vi "App - analyze RUS V6.vi"() -> ()   [LabVIEW 2015] (continued)
      w53 = FALSE  # Visible
      n14 = local read "parameters: wavepacket"() -> (w56:T16)
      n15 = local write "in sweep folder"(w57) -> ()
      n16 = call "follow the peak controller.vi"("action"=follow_the_peak_action."follow the peak", "follow the peak ref"=w50) -> ()  [unwired: 8 in, 2 out]
      n17 = property on="-- loading ..." class="Bool (strict)"("Visible"=w53) -> ()  [unwired: 2 in, 2 out]
      n18 = property on="back to temperature folder" class="Bool"("Visible"=w53) -> ()  [unwired: 2 in, 2 out]
      n19 = Bundle By Name(cluster=w56, "wavepacket is"=w52) -> (w55:T16)
      n20 = local write "parameters: wavepacket"(w55) -> ()
    }
  }
  n21 = register-events(w16, w18) -> (reference out=w48:refnum<event-registration>)  [unwired: 2 in, 1 out]
  n22 = control-ref of="save/read"() -> (w1:refnum<vi>)
  n23 = control-ref of="cursor bracket: All,  show"() -> (w19:refnum<vi>)
  n24 = control-ref of="cursor bracket: All, data window"() -> (w24:refnum<vi>)
  n25 = control-ref of="cursor bracket: All,  zoom"() -> (w23:refnum<vi>)
  n26 = control-ref of="cursor bracket: fragment"() -> (w25:refnum<vi>)
  n27 = control-ref of="cursor bracket: Time"() -> (w22:refnum<vi>)
  n28 = control-ref of="Plot: Time"() -> (w21:refnum<vi>)
  n29 = control-ref of="Plot: All"() -> (w20:refnum<vi>)
  n30 = control-ref of="Plot: fragment"() -> (w26:refnum<vi>)
  n31 = Create User Event(user event datatype=w34) -> (user event=w33:refnum<user-event>)  [unwired: 1 in, 1 out]
  n32 = Create User Event(user event datatype=w32) -> (user event=w17:refnum<user-event>)  [unwired: 1 in, 1 out]
  n33 = Create User Event(user event datatype=w47) -> (user event=w44:refnum<user-event>)  [unwired: 1 in, 1 out]
  n34 = while {
    tunnel: w48 -> [w72]
    tunnel: w16 -> [w70]
    tunnel: w44 -> [w69]
    tunnel: w36 -> [_]
    tunnel: w18 -> [w64]
    tunnel: w33 -> [w63]
    tunnel: w17 -> [w61]
    tunnel: w6 -> [w60]
    tunnel: w1 -> [w58]
    i -> [w62]
    stop <- FALSE stop-if-true
    n35 = Wait (ms)(milliseconds to wait=u32 2) -> ()  [unwired: 1 out]
    n36 = Equal To 0?(x=w62) -> ()  [unwired: 1 out]
    n37 = control-ref of="follow the peak"() -> (w59:refnum<vi>)
    n38 = event shown="[0] <calculate>: User Event" {
      selector: w72 -> [_ _ _ _ _ _ _ _ _ _]
      dyn-events: _ -> [_ _ _ _ _ _ _ _ _ _]
      timeout: 1 -> [_ _ _ _ _ _ _ _ _ _]
      tunnel: w70 -> [w98 w515 _ _ _ _ _ _ w1074 _]
      tunnel: w69 -> [_ _ _ _ _ _ _ _ _ _]
      tunnel: [_ _ _ "back to temperature folder" _ _ _ _ _ _] -> _
      tunnel: TRUE -> [w97 _ _ _ _ _ _ _ _ _]
      tunnel: FALSE -> [_ w517 _ _ w1054 _ _ _ _ _]
      tunnel: w64 -> [w100 w516 w1040 _ w1059 w1068 w1072 _ w1081 _]
      tunnel: [_ _ "Sweep folder path" _ _ _ _ _ _ _] -> _
      tunnel: w63 -> [w89 w513 _ _ _ _ _ _ _ _]
      tunnel: w61 -> [_ w491 w1038 _ _ _ _ _ _ _]
      tunnel: w60 -> [w75 _ _ _ _ _ _ _ _ _]
      tunnel: w59 -> [_ w488 _ _ _ _ _ _ _ _]
      tunnel: w58 -> [_ _ _ _ w1053 w1065 w1069 _ _ _]
      event User Event {
        w84 = FALSE  # scan/single peak
        # "all z"
        # "all omega"
        n39 = event-data() -> ("calculate"=w99:string)  [unwired: 1 in]
        n40 = local read "Sweep folder path"() -> (w81:path)
        n41 = local read "parameters: center detection"() -> (w91:T21)
        n42 = control-ref of="cursor bracket: All, data window"() -> (w95:refnum<vi>)
        n43 = local read "parameters: wavepacket"() -> (w93:T16)
        n44 = local read "parameters: omega map"() -> (w88:T22)
        n45 = local read "temperature(K)"() -> (w82:dbl)
        n46 = local read "follow the peak"() -> (w74:T7)
        n47 = control-ref of="cursor bracket: fragment"() -> (w94:refnum<vi>)
        n48 = local read "in sweep folder"() -> (w83:bool)
        n49 = local read "complex region"() -> (w90:T25)
        n50 = control-ref of="slide control"() -> (w73:refnum<vi>)
        n51 = local read "file path"() -> (w92:path)
        n52 = control-ref of="cursor bracket: All,  zoom"() -> ()  [unwired: 1 out]
        n53 = control-ref of="Plot: All"() -> (w85:refnum<vi>)
        n54 = control-ref of="cursor bracket: All,  show"() -> (w86:refnum<vi>)
        n55 = local read "plot filter progress?"() -> (w78:bool)
        n56 = Current VI's Path "Current VI's Path (this allows to inline fit function)"() -> (path=w87:path)
        n57 = control-ref of="Plot: fragment filter"() -> (w80:refnum<vi>)
        n58 = control-ref of="Plot: complex plane - filter"() -> (w79:refnum<vi>)
        n59 = for {
          N: 1 -> [_]
          tunnel: w100 -> [w131]
          tunnel: w99 -> [w130]
          tunnel: w98 -> [w129]
          tunnel: w97 -> [w126]
          shift-right: [w125] -> _
          shift-left: _ -> [w128]
          shift-right: [w124] -> _
          shift-left: _ -> [w127]
          tunnel: w95 -> [w123]
          tunnel: w94 -> [w122]
          tunnel: w93 -> [w121]
          tunnel: w92 -> [w120]
          tunnel: w91 -> [w119]
          tunnel: w90 -> [w118]
          tunnel: w89 -> [w117]
          tunnel: w88 -> [w116]
          tunnel: w87 -> [w115]
          tunnel: w86 -> [w114]
          tunnel: w85 -> [w113]
          tunnel: w84 -> [w112]
          tunnel: w83 -> [w111]
          tunnel: w82 -> [w110]
          tunnel: w81 -> [w109]
          tunnel: w80 -> [w108]
          tunnel: w79 -> [w107]
          tunnel: w78 -> [w106]
          tunnel: "filter method" -> [w105]
          tunnel: "parameters: complex fit" -> [w104]
          tunnel: w75 -> [w103]
          tunnel: w74 -> [w102]
          tunnel: w73 -> [w101]
          n60 = case shown="\"calc:peak\"" w130 {
            tunnel: w131 -> [_ _ _ w275 _ _]
            tunnel: w129 -> [_ w162 _ w268 _ w443]
            tunnel: w128 -> [w142 w151 w240 w274 w363 _]
            tunnel: w127 -> [w141 w152 w239 w273 w371 _]
            tunnel: w126 -> [_ _ _ _ _ _]
            tunnel: [w142 w151 w240 w274 w363 w442] -> w125
            tunnel: [w141 w152 w239 w273 w371 w441] -> w124
            tunnel: w123 -> [_ w148 w238 w269 w361 _]
            tunnel: w122 -> [_ _ _ w263 _ _]
            tunnel: w121 -> [w134 _ _ w264 w374 _]
            tunnel: w120 -> [_ _ _ _ _ w440]
            tunnel: w119 -> [w135 w161 _ w272 _ _]
            tunnel: w118 -> [_ _ _ _ _ _]
            tunnel: w117 -> [_ w160 _ w271 w359 _]
            tunnel: w116 -> [_ _ _ w266 _ _]
            tunnel: w115 -> [_ _ _ w270 w368 _]
            tunnel: w114 -> [_ _ _ _ w367 _]
            tunnel: w113 -> [_ _ _ w267 w353 _]
            tunnel: w112 -> [_ _ _ _ _ _]
            tunnel: w111 -> [_ _ _ w265 w360 _]
            tunnel: w110 -> [_ _ _ _ w356 _]
            tunnel: w109 -> [_ _ w218 _ _ _]
            tunnel: w108 -> [_ w159 _ _ _ _]
            tunnel: w107 -> [_ w158 _ _ _ _]
            tunnel: w106 -> [_ w157 _ _ _ _]
            tunnel: w105 -> [_ w156 _ _ _ _]
            tunnel: w104 -> [_ w143 _ w262 _ _]
            tunnel: w103 -> [_ w144 _ w261 _ _]
            tunnel: w102 -> [_ _ _ w260 _ _]
            tunnel: w101 -> [_ _ _ _ _ w435]
            frame "calc:wavepacket", Default {
              n61 = call "single fit V5.vi"("single fit parameters"=w135, "find fit action"=find_peak_action."update pond", "parameters: wavepacket"=w134) -> ("parameters: wavepacket  out"=w132:T16)  [unwired: 8 in, 4 out]
              n62 = Unbundle By Name(w132) -> ("radii vector"=w138:dbl[], "radial section"=w139:cdb[])
              n63 = Complex To Re/Im(x + iy=w139) -> (x=w137:dbl[])  [unwired: 1 out]
              n64 = local write "parameters: wavepacket"(w132) -> ()
              n65 = Bundle("radii vector"=w138, w137) -> (w136:cluster{"radii vector":dbl[], dbl[]})  [unwired: 1 in]
              n66 = Build Array(w136) -> (→"Plot: wavepacket":cluster{"radii vector":dbl[], dbl[]}[])
            }
            frame "calc:new cursor bracket" {
              n67 = call "cursor window logic V2.vi"("cursor window action"=cursor_window_action."check", "cursor window in"=w148) -> ("cursor window out"=w154:T24)  [unwired: 8 in, 1 out]
              n68 = Unbundle By Name(w154) -> ("window"=→"window":dbl)
              n69 = call "acquire cursor window data.vi"("z in"=w152, "omega in"=w151, "cursor window"=w154) -> ("z out"=w149:cdb[], "omega  out"=w150:dbl[])  [unwired: 4 in, 3 out]
              n70 = Array Size(array=w150) -> (size(s)=w147:i32)
              "# points" <- w147
              n71 = Greater?(x=w147, y=15) -> (0:w146:bool)
              n72 = case shown="True" w146 {
                tunnel: w162 -> [_ w174]
                tunnel: w161 -> [_ w173]
                tunnel: w160 -> [_ w172]
                tunnel: w159 -> [_ w171]
                tunnel: w158 -> [_ w170]
                tunnel: w157 -> [_ w169]
                tunnel: w156 -> [_ w168]
                tunnel: w150 -> [_ w167]
                tunnel: w149 -> [_ w166]
                tunnel: w144 -> [_ w165]
                tunnel: w143 -> [_ w164]
                tunnel: w143 -> [_ w163]
                frame False {
                }
                frame True {
                  n73 = flat-sequence {
                    tunnel: w173 -> [w192]
                    tunnel: w171 -> [_]
                    tunnel: w170 -> [_]
                    tunnel: w169 -> [w186]
                    tunnel: w168 -> [w185]
                    tunnel: w167 -> [w184]
                    tunnel: w166 -> [w183]
                    tunnel: w165 -> [w182]
                    tunnel: w164 -> [w181]
                    tunnel: w163 -> [_]
                    tunnel: w174 -> [w211]
                    tunnel: w172 -> [w210]
                    tunnel: [w208] -> _
                    frame #0 {
                      (unwired) TRUE
                      n74 = call "filter - complex - four.vi"("omega  in"=w184, "z in"=w183, "span"="smart filter: span", "filter method"=w185) -> ("center"=w189:cdb, "norm"=w188:dbl, "omega out"=w179:dbl[], "z in out"=w190:cdb[], "z out"=w178:cdb[], "win omega out"=w180:dbl[], "dz/domega out"=w177:cdb[], "tale of three"=w191:T38)  [unwired: 8 in]
                      "complex plane center" <- w189
                      "complex plane norm" <- w188
                      n75 = call "peak -- PM find lorenzian - V2.vi"("omega"=w179, "z"=w178, "dz/domega"=w177) -> ("phase (around center)"=w175:dbl[], "poor man lorentzian"=w176:T11)  [unwired: 9 in, 2 out]
                      n76 = case shown="True" w186 {
                        tunnel: w191 -> [_ w205]
                        tunnel: w190 -> [_ w204]
                        tunnel: w189 -> [_ w203]
                        tunnel: w188 -> [_ w202]
                        tunnel: w179 -> [_ w201]
                        tunnel: w178 -> [_ w200]
                        tunnel: w182 -> [_ w199]
                        tunnel: w181 -> [_ w198]
                        tunnel: w177 -> [_ w197]
                        tunnel: w180 -> [_ w196]
                        tunnel: w176 -> [_ w195]
                        tunnel: w175 -> [_ w194]
                        frame False {
                        }
                        frame True {
                          n77 = call "filter pipe - plot staff - more - V2.vi"("omega  in"=w201, "zin"=w204, "z out"=w200, "win omega"=w196, "phase"=w194, "dz/domega in"=w197, "center"=w203, "plots: filter related"=w199, "norm"=w202, "parameters: complex fit"=w198, "tale of three indices -- int -- control"=w205, "lorentzian"=w195) -> ()  [unwired: 8 in]
                        }
                      }
                      n78 = Bundle By Name(cluster=w192, "dz/domega"=w177, "omega in window"=w179, "z in window"=w178) -> (w193:T21)
                      n79 = local write "parameters: center detection"(w193) -> ()
                    }
                    frame #1 {
                      # "attempts at optimization :\nsmall arrays are in variables\nlarge arrays are in shift registers"
                      # "send recalculate"
                      n80 = Generate User Event(user event=w211, event data cluster="calc:peak" ("event data")) -> (error out=w209:errorcluster)  [unwired: 2 in, 1 out]
                      n81 = case shown="True" TRUE {
                        tunnel: w210 -> [_ w216]
                        tunnel: w209 -> [w212 w214]
                        tunnel: [w212 w213] -> w208
                        frame False {
                        }
                        frame True {
                          n82 = Generate User Event(user event=w216, event data cluster="check fragment zoom" ("event data"), error in=w214) -> (error out=w213:errorcluster)  [unwired: 1 in, 1 out]
                        }
                      }
                    }
                  }
                }
              }
              n83 = disable-structure shown="Disabled" {
                frame Disabled {
                  n84 = local read "interpolated gamma"() -> ()  [unwired: 1 out]
                  n85 = local read "interpolated omega"() -> ()  [unwired: 1 out]
                  n86 = local read item#-1() -> ()  [unwired: 1 out]
                }
                frame Enabled {
                }
              }
            }
            frame "save cursor window" {
              w228 = "kHz_"
              n87 = call "file -- 9w path.vi"("sweep folder"=w218) -> ("9w path"=w217:path)  [unwired: 10 in]
              n88 = call "cursor window logic V2.vi"("cursor window action"=cursor_window_action."check", "cursor window in"=w238) -> ("cursor window out"=w233:T24)  [unwired: 8 in, 1 out]
              n89 = call "acquire cursor window data.vi"("z in"=w239, "omega in"=w240, "cursor window"=w233) -> ("z out"=w222:cdb[], "omega  out"=w223:dbl[])  [unwired: 4 in, 3 out]
              n90 = Unbundle By Name(w233) -> ("left"=w232:dbl, "right"=w231:dbl)
              n91 = Number To Decimal String(number=w232) -> (decimal integer string=w230:string)  [unwired: 1 in]
              n92 = Number To Decimal String(number=w231) -> (decimal integer string=w229:string)  [unwired: 1 in]
              n93 = for {
                tunnel: w223 -> [w245] mode=indexing
                tunnel: w222 -> [w242] mode=indexing
                tunnel: [w241] -> w221 mode=indexing
                n94 = Complex To Re/Im(x + iy=w242) -> (x=w244:dbl, y=w243:dbl)
                n95 = Format Into String(format string="%f\\t%f\\t%f", w245, w244, w243) -> (resulting string=w241:string)  [unwired: 2 in, 1 out]
              }
              n96 = Strip Path(path=w217) -> (stripped path=w237:path, name=w236:string)
              n97 = call "Split file name.vi"("file name"=w236) -> ("name"=w234:string)  [unwired: 8 in, 2 out]
              n98 = Concatenate Strings(w234, "_cursor_", w230, w228, w229, w228, ".dat") -> (w226:string)
              n99 = Build Path(base path=w237, name or relative path=w226) -> (appended path=w220:path)
              n100 = call-poly <vilib>:"Write To Spreadsheet File.vi"("delimiter (\\t)"="\r", "append to file? (new file:F)"=FALSE, "1D data"=w221, "file path (dialog if empty)"=w220) -> ()  [unwired: 4 in, 1 out]
            }
            frame "calc:peak" {
              (unwired) 1
              n101 = flat-sequence {
                tunnel: w261 -> [w277]
                tunnel: w262 -> [w278]
                tunnel: w264 -> [w279]
                tunnel: w269 -> [w280]
                tunnel: w266 -> [w281]
                tunnel: w272 -> [w282]
                tunnel: [w282] -> w257
                tunnel: [w281] -> w256
                tunnel: [w280] -> w255
                tunnel: [w279] -> w254
                tunnel: [w278] -> w253
                tunnel: [w277] -> w252
                tunnel: [w276] -> w250
                tunnel: w270 -> [_]
                tunnel: w263 -> [w295]
                tunnel: w267 -> [w299]
                tunnel: [w294] -> w259
                tunnel: w260 -> [w289]
                tunnel: w257 -> [w304]
                tunnel: w256 -> [w301]
                tunnel: w255 -> [w298]
                tunnel: w254 -> [w292]
                tunnel: w253 -> [w291]
                tunnel: w252 -> [w290]
                tunnel: [w286] -> w251
                tunnel: w250 -> [w286]
                tunnel: "Use C++" -> [w285]
                tunnel: "find fit action" -> [w284]
                tunnel: "plot pm ?" -> [w283]
                tunnel: w259 -> [w334]
                tunnel: [w334] -> w258
                tunnel: w251 -> [w332]
                tunnel: w275 -> [w341]
                tunnel: w265 -> [w340]
                tunnel: w271 -> [w339]
                tunnel: w268 -> [w338]
                tunnel: w258 -> [w335]
                frame #0 {
                  n102 = Tick Count (ms)() -> (millisecond timer value=w276:u32)
                }
                frame #1 {
                  n103 = case shown="True" w285 {
                    tunnel: w304 -> [w317 w330]
                    tunnel: [w316 w329] -> w303
                    tunnel: [w315 w328] -> w302
                    tunnel: w301 -> [w314 w327]
                    tunnel: [w313 w326] -> w300
                    tunnel: [w312 w325] -> w297
                    tunnel: w295 -> [w311 w324]
                    tunnel: w284 -> [w310 w323]
                    tunnel: [w309 w322] -> w293
                    tunnel: w292 -> [w308 w321]
                    tunnel: w291 -> [w307 w320]
                    tunnel: w290 -> [w306 w319]
                    tunnel: w283 -> [w305 w318]
                    frame True {
                      n104 = call "single fit V5cpp.vi"("single fit parameters"=w317, "plot what"=w305, "find fit action"=w310, "cursor bracket: fragment  ref"=w311, "omega map parameters"=w314, "parameters: wavepacket"=w308, "parameters: complex fit"=w307, "plots: filter related"=w306) -> ("single fit parameters out"=w316:T21, "omega map parameters out"=w315:T22, "parameters: wavepacket  out"=w309:T16, "complex region out"=w313:T25, "lorentzian out"=w312:T11)  [unwired: 3 in]
                    }
                    frame False {
                      n105 = call "single fit V5.vi"("single fit parameters"=w330, "plot what"=w318, "find fit action"=w323, "cursor bracket: fragment  ref"=w324, "omega map parameters"=w327, "parameters: wavepacket"=w321, "parameters: complex fit"=w320, "plots: filter related"=w319) -> ("single fit parameters out"=w329:T21, "omega map parameters out"=w328:T22, "parameters: wavepacket  out"=w322:T16, "complex region out"=w326:T25, "lorentzian out"=w325:T11)  [unwired: 3 in]
                    }
                  }
                  n106 = local write "parameters: center detection"(w303) -> ()
                  n107 = local write "parameters: wavepacket"(w293) -> ()
                  n108 = local write "parameters: omega map"(w302) -> ()
                  n109 = call "shake it.vi"("cursor bracket : fragment 2"=w295, "cursor bracket: All, data window 2"=w298, "Plot: All"=w299, "follow the peak Con"=w289, "search attempts"=4, "peak close to center -- factor"=0.3, "lorentzian"=w297) -> ("Boolean"=w294:bool, "lorentzian out"=w296:T11)  [unwired: 1 in, 2 out]
                  n110 = local write "complex region"(w300) -> ()
                  n111 = local write "lorentzian"(w296) -> ()
                }
                frame #2 {
                  n112 = Tick Count (ms)() -> (millisecond timer value=w333:u32)
                  n113 = Subtract(x=w333, y=w332) -> (x-y=→"fit time (ms)":u32)
                }
                frame #3 {
                  n114 = case shown="True" w335 {
                    tunnel: w341 -> [_ w348]
                    tunnel: w340 -> [_ w347]
                    tunnel: w339 -> [_ w346]
                    tunnel: w338 -> [w343 _]
                    tunnel: [w343 w345] -> w337
                    tunnel: ["calc:new cursor bracket" ("t.folder") w344] -> w336
                    frame False {
                    }
                    frame True {
                      n115 = case shown="True" w347 {
                        tunnel: w348 -> [_ w352]
                        tunnel: w346 -> [w350 _]
                        tunnel: [w350 w352] -> w345
                        tunnel: ["calculation finished" ("t.folder") "update freq/atten" ("t.folder")] -> w344
                        frame False {
                        }
                        frame True {
                        }
                      }
                    }
                  }
                  n116 = Generate User Event(user event=w337, event data cluster=w336) -> ()  [unwired: 2 in, 2 out]
                }
              }
            }
            frame "calc: scan" {
              n117 = property class="Clust (strict)"(reference=w361) -> ("Value"=w366:T39)  [unwired: 1 in, 2 out]
              n118 = Unbundle By Name(w366) -> ("left"=w365:dbl, "right"=w364:dbl)
              n119 = Array Size(array=w371) -> (size(s)=w373:i32)
              n120 = call "index from range.vi"("left"=w365, "right"=w364, "omega"=w363) -> ("length"=w362:dbl)  [unwired: 6 in, 2 out]
              n121 = Quotient & Remainder(x=w373, y="scan speed") -> (floor(x/y)=w372:i32)  [unwired: 1 out]
              n122 = for {
                N: w372 -> [_]
                tunnel: w374 -> [w425]
                tunnel: w363 -> [w423]
                tunnel: w371 -> [w433]
                shift-right: [w422] -> _
                shift-left: 0 -> [w414]
                tunnel: "scan speed" -> [w432]
                tunnel: w368 -> [w431]
                tunnel: w367 -> [_]
                tunnel: w353 -> [w416]
                tunnel: w362 -> [w411]
                tunnel: w361 -> [w412]
                tunnel: [w405] -> w357
                tunnel: "number of hits to threshold" -> [w407]
                tunnel: "threshold window" -> [w406]
                i -> [w434]
                n123 = Add(x=w414, y=w432) -> (x+y=w422:i32)
                n124 = Equal To 0?(x=w434) -> (x = 0?=w408:bool)
                n125 = Subtract(x=w414, y=w411) -> (x-y=w413:dbl)
                n126 = Array Subset(array=w423, index=w414, length=w432) -> (w429:dbl[])
                n127 = Index Array(array=w423, index #1=w414, index #2=w413) -> (element #1=w421:dbl, element #2=w420:dbl)
                n128 = Array Subset(array=w433, index=w414, length=w432) -> (w430:cdb[])
                n129 = Subtract(x=w420, y=w421) -> ()  [unwired: 1 out]
                n130 = Add(x=w421, y=w420) -> (x+y=w419:dbl)
                n131 = Divide(x=w419, y=2) -> (x/y=w409:dbl)
                n132 = call "curvature-cator - ia.vi"("omega array in"=w429, "size"=w411, "number of grid points"=70, "decimation threshold"=1, "z array in"=w430, "wavepacket in"=w425, "scale factor"=3.0, "first time"=w408, "main VI path"=w431) -> ("lorentzian out"=w424:T11)  [unwired: 3 in, 3 out]
                n133 = call "cursor window logic V2.vi"("cursor window action"=cursor_window_action."change center", "center"=w409, "cursor window in"=w412) -> ("cursor window out"=w403:T24)  [unwired: 7 in, 1 out]
                n134 = Unbundle By Name(w424) -> ("omega(0)"=w396:dbl)  [unwired: 1 out]
                n135 = call "aggregator - i.vi"("requested averaging interval"=10, "first time"=w408, "requested size"=w411, "number"=w396) -> ()  [unwired: 3 in, 5 out]
                n136 = call "aggregator - i.vi"("first time"=w408, "requested size"=w411, "number"=w409) -> ()  [unwired: 4 in, 5 out]
                n137 = Unbundle By Name(w403) -> ("left"=w402:dbl, "right"=w401:dbl)
                n138 = call "Q -- check range.vi"("upper"=w401, "lower"=w402, "number"=w396) -> ("in range?"=w397:bool)  [unwired: 4 in, 4 out]
                n139 = Select(t=w396, s=w397, f=nan ("scale factor")) -> (s? t:f=w394:dbl)
                n140 = call "threshold-icator - i.vi"("first time"=w408, "requested size"=w407, "gamma"=w406, "omega"=w394) -> ("new peak"=w393:bool, "array of peaks"=w405:dbl[])  [unwired: 3 in, 3 out]
                "array of peaks" <- w405
                n141 = Select(t=u32 327424 ("Color Box"), s=w393, f=u32 16716367 ("Color Box")) -> (s? t:f=w398:u32)
                n142 = call "replace cursor - plot ref.vi"("cursor state"=T35."colored", "Color Box"=w398, "action"=enum16{"", "read", "write"}."write" ("Enum"), "cursor index"=9, "new X"=w396, "Plot ref in"=w416) -> ()  [unwired: 3 in, 3 out]
              }
              n143 = case shown="True" w360 {
                selector: w360 -> [_ w379]
                tunnel: w359 -> [_ w385]
                tunnel: "calculation finished" ("t.folder") -> [_ w384]
                tunnel: w357 -> [_ w383]
                tunnel: w356 -> [_ w382]
                frame False {
                }
                frame True {
                  n144 = call "switch - C.vi"("switch"=w379) -> ("result"=w378:bool)  [unwired: 10 in]
                  n145 = for {
                    tunnel: w383 -> [w391] mode=indexing
                    tunnel: w382 -> [w390]
                    tunnel: [w389] -> w376
                    tunnel: [w388] -> w375
                    tunnel: w378 -> [w387]
                    tunnel: 50000 -> [w386]
                    n146 = call "aggregator.vi"("first time"=w387, "requested size"=w386, "number"=w390) -> ("Array"=w388:cdb[])  [unwired: 8 in]
                    n147 = call "aggregator.vi"("first time"=w387, "requested size"=w386, "number"=w391) -> ("Array"=w389:cdb[])  [unwired: 8 in]
                  }
                  n148 = Bundle("Array"=w375, "Array"=w376) -> (w381:cluster{"Array":cdb[], "Array":cdb[]})  [unwired: 1 in]
                  n149 = Build Array(w381) -> (→"Plot: JBBetts":cluster{"Array":cdb[], "Array":cdb[]}[])
                  n150 = Generate User Event(user event=w385, event data cluster=w384) -> ()  [unwired: 2 in, 2 out]
                }
              }
            }
            frame "calc:new file" {
              n151 = flat-sequence {
                tunnel: w440 -> [w447]
                tunnel: [w447] -> w439
                tunnel: [w446] -> w437
                tunnel: [w463] -> w445
                tunnel: [w462] -> w444
                tunnel: w439 -> [w464]
                tunnel: w435 -> [w451]
                tunnel: [w483] -> w441
                tunnel: [w484] -> w442
                tunnel: w445 -> [w484]
                tunnel: w444 -> [w483]
                tunnel: w443 -> [w482]
                tunnel: [w480] -> w438
                frame #0 {
                  n152 = Tick Count (ms)() -> (millisecond timer value=w446:u32)
                }
                frame #1 {
                  # "Hz/kHz"
                  n153 = local read "plot fit progress?"() -> (w457:bool)
                  n154 = call "slide controller.vi"("slide action"=slide_action."check", "slide control"=w451) -> ("in slide"=w449:bool)  [unwired: 6 in, 3 out]
                  n155 = Not(x=w457) -> (.not. x?=w459:bool)
                  n156 = And(x=w459, y=w449) -> (x .and. y?=w458:bool)
                  n157 = call "rus fit - load data file.vi"("file path"=w464, "read scan file"="read scan file options") -> ("all:max omega"=→"all:max omega":dbl, "all:min omega"=→"all:min omega":dbl, "omega"=w463:dbl[], "x + iy"=w462:cdb[])  [unwired: 5 in, 1 out]
                  n158 = Not(x=w458) -> (.not. x?=w456:bool)
                  n159 = control-ref of="Plot: All"() -> (w453:refnum<vi>)
                  n160 = case shown="True" w456 {
                    tunnel: w463 -> [_ w474]
                    tunnel: w462 -> [_ w473]
                    frame False {
                    }
                    frame True {
                      n161 = Complex To Re/Im(x + iy=w473) -> (x=w476:dbl[], y=w475:dbl[])
                      n162 = Bundle("omega"=w474, w476) -> (w477:cluster{"omega":dbl[], dbl[]})  [unwired: 1 in]
                      n163 = Bundle("omega"=w474, w475) -> (w478:cluster{"omega":dbl[], dbl[]})  [unwired: 1 in]
                      n164 = Build Array(w477, w478) -> (→"Plot: All":cluster{"omega":dbl[], dbl[]}[])
                    }
                  }
                  n165 = case shown="\"log-log\"" "mapping: All" {
                    tunnel: [u8 0 ("X Scale.Mapping Mode") u8 1 ("X Scale.Mapping Mode") u8 0 ("X Scale.Mapping Mode") u8 1 ("X Scale.Mapping Mode")] -> w455
                    tunnel: [u8 0 ("X Scale.Mapping Mode") u8 0 ("X Scale.Mapping Mode") u8 1 ("X Scale.Mapping Mode") u8 1 ("X Scale.Mapping Mode")] -> w452
                    frame "linear-linear", Default {
                    }
                    frame "log-linear" {
                    }
                    frame "linear-log" {
                    }
                    frame "log-log" {
                    }
                  }
                  n166 = property on="Property Node" class="XYGraph (strict)"(reference=w453, "XScale.Mapping Mode"=w455, "YScale.Mapping Mode"=w452) -> ()  [unwired: 1 in, 2 out]
                }
                frame #2 {
                  n167 = Tick Count (ms)() -> (millisecond timer value=w480:u32)
                  n168 = Generate User Event(user event=w482, event data cluster="calc:new cursor bracket" ("event data")) -> ()  [unwired: 2 in, 2 out]
                }
              }
              n169 = Subtract(x=w438, y=w437) -> (x-y=→"ms per read":u32)
            }
          }
        }
      }
      event User Event {
        # "Temperature folder logic:\nwe load the whole folder (temperatures, timestamps,  paths -- not the data) in \"sweep folder file path array\".\nFiles are  navigated by using \"time (min)\" variable. The lorentzian fits are stored in \n\"frequency points\", \"attenuation points\" etc arrays and are displayed in plots.\n\nWhen we read a single file the variable \"in temperature folder\" is FALSE  and nothing of the above (and below) applies"
        n170 = event-data() -> ("temperature folder control"=w510:string)  [unwired: 1 in]
        n171 = local read "t.folder file path array"() -> (w499:T26[])
        n172 = local read "cursor bracket: Time"() -> (w502:T24)
        n173 = local read "temperature points"() -> (w500:dbl[])
        n174 = local read "best fit parameters"() -> (w494:dbl[])
        n175 = local read "attenuation points"() -> (w486:dbl[])
        n176 = local read "Sweep folder path"() -> (w511:path)
        n177 = local read "Magn Field points"() -> (w485:dbl[])
        n178 = local read "frequency points"() -> (w490:dbl[])
        n179 = local read "lorentzian points"() -> (w497:T27[])
        n180 = local read "in sweep folder"() -> (w509:bool)
        n181 = local read "9w folder path"() -> (w505:path)
        n182 = local read "time points"() -> (w501:dbl[])
        n183 = local read "lorentzian"() -> (w503:T11)
        n184 = local read "file path"() -> (w504:path)
        n185 = local read "fit using"() -> (w493:T5)
        n186 = control-ref of="Plot: Time"() -> (w496:refnum<vi>)
        n187 = local read "tfolder"() -> (w498:T30)
        n188 = control-ref of="cursor bracket: Time"() -> (w489:refnum<vi>)
        n189 = control-ref of="save/read"() -> (w487:refnum<vi>)
        n190 = control-ref of="cursor bracket: Time"() -> (w508:refnum<vi>)
        n191 = control-ref of="cursor bracket: All, data window"() -> (w507:refnum<vi>)
        n192 = control-ref of="cursor bracket: All,  zoom"() -> ()  [unwired: 1 out]
        n193 = control-ref of="cursor bracket: fragment"() -> (w506:refnum<vi>)
        n194 = case shown="\"new temperature folder\"" w510 {
          tunnel: w511 -> [w521 _ _ _ _ _ w690 w715 _ _ _ _ _ _ _ _ _]
          tunnel: TRUE -> [w530 _ _ _ _ _ _ w709 _ _ _ _ _ _ _ _ _]
          tunnel: w517 -> [_ _ _ _ _ _ _ _ _ w821 _ _ _ _ _ _ _]
          tunnel: w516 -> [_ _ _ _ w581 _ _ w720 _ _ _ _ w994 _ _ _ w1028]
          tunnel: w515 -> [_ _ _ _ w582 w637 _ _ _ _ _ w930 _ _ w1010 _ _]
          tunnel: FALSE -> [_ _ _ _ _ _ _ _ w810 _ _ _ _ _ _ _ _]
          tunnel: w513 -> [_ _ _ _ _ _ _ _ _ w820 _ _ _ _ _ _ _]
          tunnel: 0 -> [w529 _ _ _ _ _ _ _ _ _ _ _ _ _ _ _ _]
          tunnel: w509 -> [w528 _ w562 w564 w584 w639 w692 _ _ w813 w877 w923 _ _ _ _ _]
          tunnel: w499 -> [_ _ _ _ _ _ _ _ _ _ _ w929 _ _ _ _ _]
          tunnel: w508 -> [_ _ _ _ _ _ _ w713 _ _ _ _ _ _ _ _ _]
          tunnel: w498 -> [w520 _ _ _ _ _ _ w712 _ _ _ _ _ _ _ _ _]
          tunnel: w507 -> [_ _ _ _ w583 w638 _ _ _ _ _ w928 _ _ w1011 _ _]
          tunnel: w506 -> [_ _ _ _ _ _ _ _ _ _ _ w927 _ _ _ _ _]
          tunnel: w505 -> [_ _ w559 _ w587 w643 w694 _ _ _ _ _ _ _ _ _ _]
          tunnel: w504 -> [_ _ w561 _ _ _ _ _ _ _ _ _ _ _ _ _ _]
          tunnel: w503 -> [_ _ w557 _ _ _ w693 _ _ w819 _ w925 _ _ w1012 _ _]
          tunnel: w502 -> [w526 _ _ w569 _ w642 _ _ _ _ _ _ _ _ _ _ _]
          tunnel: w501 -> [w527 _ _ w565 w585 w640 _ _ _ w818 _ w926 w998 _ _ _ w1033]
          tunnel: w500 -> [_ _ _ w566 w586 w641 _ _ _ w817 w879 _ w999 _ _ _ w1032]
          tunnel: w497 -> [w525 _ _ _ _ _ _ _ _ w816 w878 _ _ _ _ _ _]
          tunnel: w496 -> [_ _ _ _ _ _ _ w711 _ _ _ w924 _ _ _ _ w1029]
          tunnel: "monotonic segment" -> [_ _ _ _ _ _ _ w710 _ _ _ _ _ _ _ _ _]
          tunnel: w494 -> [w524 _ _ _ _ _ _ _ _ w815 _ _ _ _ _ _ _]
          tunnel: w493 -> [w522 _ _ w568 _ _ _ _ _ w814 _ _ _ _ _ _ _]
          tunnel: "varshni win (relative)" -> [w523 _ _ w567 _ _ _ _ _ _ _ _ _ _ _ _ _]
          tunnel: w491 -> [_ _ _ _ _ _ _ w708 _ _ _ _ _ _ _ _ _]
          tunnel: w490 -> [_ _ _ w563 _ w636 _ _ _ _ _ _ _ _ _ _ _]
          tunnel: w489 -> [_ _ _ _ _ _ _ _ _ _ _ _ w1002 _ _ _ _]
          tunnel: w486 -> [_ _ _ _ _ w635 _ _ _ _ _ _ _ _ _ _ _]
          tunnel: w488 -> [_ _ _ _ _ _ _ w707 _ _ _ w922 _ w1005 _ _ _]
          tunnel: w487 -> [w519 _ _ _ w580 w634 w691 w706 _ w812 _ _ _ _ w1009 w1023 _]
          tunnel: w485 -> [_ _ _ _ _ _ _ _ _ w811 w876 _ w993 _ _ _ w1026]
          frame "write freq file", Default {
            n195 = case shown="True" w528 {
              tunnel: w530 -> [_ _]
              tunnel: w529 -> [_ w550]
              tunnel: w520 -> [_ w549]
              tunnel: w527 -> [_ w547]
              tunnel: w526 -> [_ _]
              tunnel: w525 -> [_ w548]
              tunnel: w524 -> [_ _]
              tunnel: w523 -> [_ w546]
              tunnel: w522 -> [_ w545]
              tunnel: w521 -> [_ w536]
              tunnel: w519 -> [_ w534]
              frame False {
              }
              frame True {
                (unwired) 1.2 ("Varshni win(kHz)")
                (unwired) FALSE
                # "black - file is written - OK\nred -- arrays changed since last save -- set in update freq/atten"
                # "file is always <t.folder.path>/../9w/<name>.dat"
                n196 = local write "to a file: used counter"(w550) -> ()
                n197 = call "file -- 9w path.vi"("sweep folder"=w536) -> ("9w path"=w535:path)  [unwired: 10 in]
                n198 = call "freq file read-write controller.vi"("action"=save-read_action."saved file clean", "save/read"=w534) -> ("save read out"=w532:T6)  [unwired: 7 in, 2 out]
                n199 = call "file -- open-create folder.vi"("folder name"="backup" ("name or relative path"), "base path"=w535) -> ("folder path out"=w537:path)  [unwired: 9 in]
                n200 = call "file -- open-create folder.vi"("folder name"="segments" ("name or relative path"), "base path"=w535) -> ("folder path out"=w539:path)  [unwired: 9 in]
                n201 = Unbundle By Name(w532) -> ("to a file"=w531:string)
                n202 = Concatenate Strings(w531, ".dat" ("name or relative path")) -> (w541:string)
                n203 = Build Path(base path=w535, name or relative path=w541) -> (appended path=w544:path)
                "freqout file" <- w544
                n204 = call "rus fit - write freqout file.vi"("time points"=w547, "Varshni win(relative)"=w546, "to a file"=w531, "fit using"=w545, "segments folder"=w539, "freqout file"=w544, "tfolder"=w549, "lorentzian pts"=w548) -> ()  [unwired: 4 in]
                n205 = call <vilib>:"Check if File or Folder Exists.vi"("path"=w544) -> ("file or folder exists?"=w543:bool, "dup path"=w542:path)  [unwired: 8 in, 1 out]
                n206 = case shown="True" w543 {
                  tunnel: w542 -> [_ w556]
                  tunnel: w541 -> [_ w555]
                  tunnel: w537 -> [_ w554]
                  frame False {
                  }
                  frame True {
                    n207 = Build Path(base path=w554, name or relative path=w555) -> (appended path=w553:path)
                    n208 = Copy(9:TRUE ("overwrite (F)"), 10:w553, 11:w556) -> ()  [unwired: 2 in, 3 out]
                  }
                }
              }
            }
          }
          frame "empty" {
          }
          frame "write RPR line" {
            n209 = Strip Path(path=w561) -> (stripped path=w560:path)  [unwired: 1 out]
            n210 = Select(t=w559, s=w562, f=w560) -> (s? t:f=w558:path)
            n211 = call "rus fit - write RPR line.vi"("folder path"=w558, "lorentzian"=w557) -> ()  [unwired: 10 in]
          }
          frame "update delta freq" {
            n212 = case shown="True" w564 {
              tunnel: w569 -> [_ w579]
              tunnel: w568 -> [_ w573]
              tunnel: w567 -> [_ w578]
              tunnel: w566 -> [_ w571]
              tunnel: w565 -> [_ w572]
              tunnel: w563 -> [_ w570]
              frame False {
              }
              frame True {
                n213 = call "fit -- freq vs T controller.vi"("time points"=w572, "varshni win (relative)"=w578, "fit using"=w573, "temperature points"=w571, "frequency points"=w570, "cursor bracket: Time"=w579) -> ("best fit parameters"=→"best fit parameters":dbl[], "fit function name"=→"fit function name":string, "fit points before"=→"fit points before":i32, "fit points after"=→"fit points after":i32)  [unwired: 6 in]
              }
            }
          }
          frame "read freq file" {
            n214 = case shown="True" w584 {
              selector: w584 -> [_ w598]
              tunnel: w587 -> [_ w611]
              tunnel: w586 -> [_ w610]
              tunnel: w585 -> [_ w603]
              tunnel: w583 -> [_ _]
              tunnel: w582 -> [_ _]
              tunnel: w581 -> [_ w599]
              tunnel: w580 -> [_ w592]
              frame False {
              }
              frame True {
                w600 = "set data win to extrapolated time"  # event data
                n215 = call "freq file read-write controller.vi"("action"=save-read_action."check", "save/read"=w592) -> ("save read out"=w590:T6, "save/read OUT"=w588:refnum<vi>)  [unwired: 7 in, 1 out]
                n216 = Unbundle By Name(w590) -> ("from file"=w589:string)
                n217 = Concatenate Strings(w589, ".dat" ("name or relative path")) -> (w616:string)
                n218 = Array Max & Min(array=w603) -> (max value=w605:dbl, min value=w604:dbl)  [unwired: 2 out]
                n219 = local read "attenuation points"() -> (w607:dbl[])
                n220 = local read "frequency points"() -> (w608:dbl[])
                n221 = local read "lorentzian points"() -> (w609:T27[])
                n222 = Build Path(base path=w611, name or relative path=w616) -> (appended path=w614:path)
                n223 = call <vilib>:"Check if File or Folder Exists.vi"("path"=w614) -> ("file or folder exists?"=w595:bool, "dup path"=w613:path)  [unwired: 8 in, 1 out]
                n224 = Generate User Event(user event=w599, event data cluster=w600) -> ()  [unwired: 2 in, 2 out]
                n225 = Select(t=save-read_action."read file OK" ("action"), s=w595, f=save-read_action."read file not OK" ("action")) -> (s? t:f=w594:T36)
                n226 = And(x=w595, y=w598) -> (x .and. y?=w612:bool)
                n227 = call "freq file read-write controller.vi"("action"=w594, "save/read"=w588) -> ("save/read OUT"=w593:refnum<vi>)  [unwired: 7 in, 2 out]
                n228 = case shown="True" w612 {
                  tunnel: w613 -> [_ w633]
                  tunnel: w604 -> [_ w630]
                  tunnel: w605 -> [_ w629]
                  tunnel: w603 -> [_ w632]
                  tunnel: w610 -> [_ w631]
                  tunnel: w609 -> [w621 w628]
                  tunnel: w608 -> [w620 w627]
                  tunnel: w607 -> [w619 w626]
                  tunnel: [w621 w625] -> w606
                  tunnel: [w620 w624] -> w602
                  tunnel: [w619 w623] -> w601
                  frame False {
                  }
                  frame True {
                    n229 = call "rus fit - read freq file.vi"("temperature points IN"=w631, "right"=w629, "time points IN"=w632, "left"=w630, "file path"=w633, "attenuation points IN"=w626, "frequency points IN"=w627, "lorentzian points IN"=w628) -> ("format version"=→"format version":string, "attenuation points OUT"=w623:dbl[], "frequency points OUT"=w624:dbl[], "lorentzian points OUT"=w625:T27[])
                  }
                }
                n230 = case shown="True" w595 {
                  tunnel: w593 -> [_ w618]
                  frame False {
                  }
                  frame True {
                    n231 = call "freq file read-write controller.vi"("action"=save-read_action."copy read to save", "save/read"=w618) -> ()  [unwired: 7 in, 3 out]
                  }
                }
                n232 = local write "attenuation points"(w601) -> ()
                n233 = local write "lorentzian points"(w606) -> ()
                n234 = local write "frequency points"(w602) -> ()
              }
            }
          }
          frame "set data win to extrapolated time" {
            # "input is full file path"
            n235 = case shown="True" w639 {
              tunnel: w643 -> [_ _]
              tunnel: w642 -> [_ _]
              tunnel: w641 -> [_ _]
              tunnel: w640 -> [_ w674]
              tunnel: w638 -> [_ w670]
              tunnel: w637 -> [_ w669]
              tunnel: w636 -> [_ w652]
              tunnel: w635 -> [_ w663]
              tunnel: w634 -> [_ w657]
              frame False {
              }
              frame True {
                w661 = "calc:new cursor bracket"  # event data
                n236 = local read "time (min)"() -> (w673:dbl)
                n237 = Threshold 1D Array(2:w673, 3:w674) -> (0:w647:dbl)  [unwired: 1 in]
                n238 = call "freq file read-write controller.vi"("action"=save-read_action."check", "save/read"=w657) -> ("save read out"=w655:T6)  [unwired: 7 in, 2 out]
                n239 = Unbundle By Name(w655) -> ("from file"=w654:string)
                n240 = Decimal String To Number(string=w654) -> (number=w653:i32)  [unwired: 2 in, 1 out]
                n241 = Split 1D Array(array=w652, index=w647) -> (first subarray=w651:dbl[], second subarray=w649:dbl[])
                n242 = for {
                  tunnel: w649 -> [w683] mode=indexing
                  tunnel: [w681] -> w646
                  i -> [w681]
                  stop <- w682 stop-if-true
                  n243 = Greater Than 0?(x=w683) -> (x > 0?=w682:bool)
                }
                n244 = Reverse 1D Array(array=w651) -> (reversed array=w650:dbl[])
                n245 = for {
                  tunnel: w650 -> [w686] mode=indexing
                  tunnel: [w684] -> w644
                  i -> [w684]
                  stop <- w685 stop-if-true
                  n246 = Greater Than 0?(x=w686) -> (x > 0?=w685:bool)
                }
                n247 = Greater Or Equal?(x=w644, y=w646) -> (x >= y?=w648:bool)
                n248 = case shown="False" w648 {
                  tunnel: w647 -> [w677 w680]
                  tunnel: w646 -> [_ w679]
                  tunnel: [w675 w678] -> w645
                  tunnel: w644 -> [w676 _]
                  frame False {
                    n249 = Subtract(x=w677, y=w676) -> (x-y=w675:dbl)
                  }
                  frame True {
                    n250 = Add(x=w680, y=w679) -> (x+y=w678:dbl)
                  }
                }
                n251 = Index Array(array=w663, index=w645) -> (element=w668:dbl)
                n252 = Index Array(array=w652, index=w645) -> (element=w672:dbl)
                n253 = call "Q -- check range -- i -- real.vi"("lower"=1.0, "number"=w672) -> ("in range?"=w660:bool, "number in range"=w659:dbl)  [unwired: 7 in, 1 out]
